vi "buildColorArray_test.vi"() -> ()   [LabVIEW 2014]
uses:
  DataTypes/DataTypes.llb/Indexes.ctl
panel:
  out "output array":u32[](array[numeric])
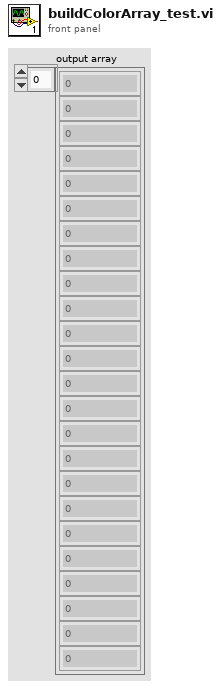
[diagram p1: front panel]
types:
  T1 = typedef "Indexes.ctl" = cluster{"BASE COLOR":dbl[], "COLOR1":dbl[], "COLOR2":dbl[], "COLOR3":dbl[], "COLOR4":dbl[], "COLOR5":dbl[]}
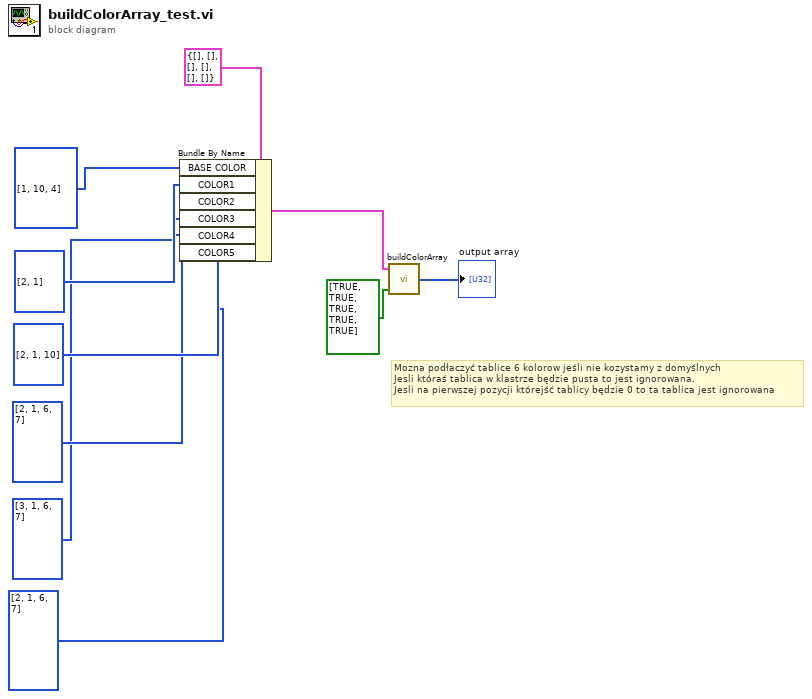
[diagram p0: block diagram]
diagram:
  # "Mozna podłaczyć tablice 6 kolorow jeśli nie kozystamy z domyślnych\nJesli któraś tablica w klastrze będzie pusta to jest ignorowana.\nJesli na pierwszej pozycji którejść tablicy będzie 0 to ta tablica jest ignorowana"
  n1 = Bundle By Name(cluster=T1 {"BASE COLOR"=[], "COLOR1"=[], "COLOR2"=[], "COLOR3"=[], "COLOR4"=[], "COLOR5"=[]} ("Color Lists"), "BASE COLOR"=i32[] [1, 10, 4], "COLOR1"=i32[] [2, 1], "COLOR2"=i32[] [2, 1, 10], "COLOR3"=i32[] [2, 1, 6, 7], "COLOR4"=i32[] [3, 1, 6, 7], "COLOR5"=i32[] [2, 1, 6, 7]) -> (w4:T1)
  n2 = call "buildColorArray.vi"("Array"=bool[] [TRUE, TRUE, TRUE, TRUE, TRUE], "Color Lists"=w4) -> ("output array"=→"output array":u32[])  [unwired: 1 in]
